vi "Barcode Detector.vi"() -> ()   [LabVIEW 2017]
uses:
  IMAQCV/PIIO.lvlib
  IMAQCV/GPIO/GPIO Pins.ctl
  IMAQCV/IMAQCV.lvlib
  IMAQCV/LVOpenCV.lvlib
  <vilib>/Platform/TimedLoop/XDataNode/wakeup.ctl
  <vilib>/Platform/TimedLoop/XDataNode/XDNodeRunTimeDep.lvlib
  <vilib>/Platform/TimedLoop/XDataNode/nitl_modes.ctl
  <vilib>/Platform/TimedLoop/XDataNode/timing_clust.ctl
  <vilib>/platform/TimedLoop/XDataNode/XDataNode.xnode
  IMAQCV/Support/Camera.ctl
panel:
  out "Barcode":string[](array[string])
  out "output per minute":u32
  in  "FPS":i32=30
  in  "RGB LED 8x8":u32[][](array[colorbox])=[[0, 0, 16777215, 16777215, 16777215, 16777215, 16777215, 16777215], [0, 16777215, 16777215, 16777215, 16777215, 16777215, 16777215, 16777215], [16777215, 16777215, 16777215, 16777215, 16777215, 16777215, 16777215, 16777215], [16777215, 16777215, 0, 0, 0, 0, 0, 0], [16777215, 16777215, 0, 0, 0, 0, 0, 0], [16777215, 16777215, 0, 0, 0, 0, 0, 0], [16777215, 16777215, 0, 0, 0, 0, 0, 0], [0, 16777215, 16777215, 16777215, 16777215, 0, 0, 0]]
  in  "PIN":u8(ring)=23 items=["DIO9"=19, "DIO10"=18, "DIO11"=17, "DIO12"=16, "DIO13"=15, "DIO14"=14, "DIO15"=21, "DIO16"=20, "DIO17"=0, "DIO18"=1, "DIO19"=2, "DIO20"=3, "DIO21"=5, "DIO22"=6, "DIO23"=9, "SDA"=22, "SCL"=23]
  in  "camera input":T1=enum."USB1"
  in  "Image Size":T2(ring)=enum."640 (H)   x  480 (V) "
  out "picture":picture
  out "image processing time (ms)":u32
  out "IO8":bool
  out "IO7":bool
  out "IO6":bool
  out "IO5":bool
  out "IO4":bool
  out "IO3":bool
  out "IO2":bool
  in  "delay (ms)":u32=150
  out "moving time (ms)":u32
  in  "LED Flash":bool
  in  "LED":bool
  in  "Gain (0=auto)":i32(slide) scale=0.0..100.0
  in  "Brightness":i32(slide)=50 scale=0.0..100.0
  in  "Contrast":i32(slide)=50 scale=0.0..100.0
  in  "Saturation":i32(slide)=50 scale=0.0..100.0
  in  "Sharpness":i32(slide)=50 scale=0.0..100.0
  in  "Rotation":i32(ring) items=["0", "90", "180", "270"]
  in  "Flip Horizontal":bool
  in  "Flip Vertical":bool
  in  "AWB":T3(ring)
  in  "Meter":enum16{"AVERAGE", "SPOT", "BACKLIT", "MATRIX"}(ring)
  in  "Effect":T4(ring)
  in  "Shutter (us, 0=auto)":i32
  out "IO1":bool
  in  "stop":bool
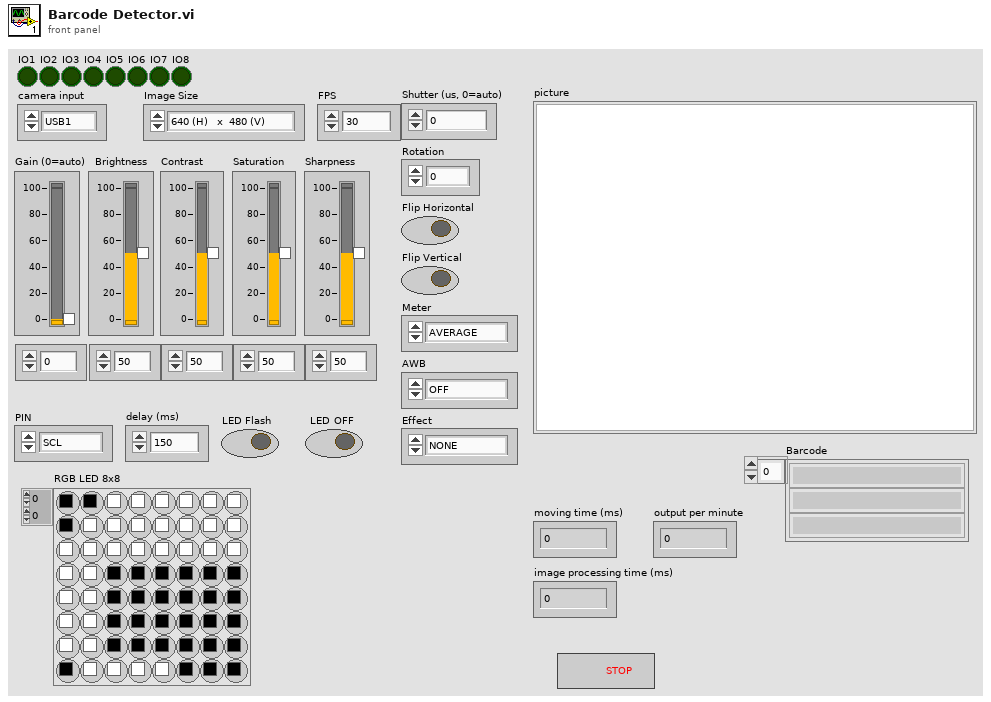
[diagram p1: front panel]
types:
  T1 = typedef "IMAQCV.lvlib/Camera.ctl" = enum8{"Picam", "USB1", "USB2", "USB3", "USB4"}
  T2 = enum16{"320 (H)   x  240 (V)", "352(H)    x  288 (V)", "640 (H)   x  480 (V) ", "800 (H)   x  600 (V)", "1024 (H) x  768 (V)", "1280 (H) x  720 (V)", "1280 (H) x  960 (V)", "1280 (H) x 1024 (V)", "1920 (H) x 1080 (V)"}
  T3 = enum16{"OFF", "AUTO", "SUNLIGHT", "CLOUDY", "SHADE", "TUNGSTEN", "FLUORESCENT", "INCANDESCENT", "FLASH"}
  T4 = enum16{"NONE", "NEGATIVE", "SOLARIZE", "SKETCH", "DENOISE", "EMBOSS", "OILPAINT", "HATCH", "GPEN", "PASTEL", "WATERCOLOR", "FILM", "BLUR", "SATURATION", "COLORSWAP", "WASHEDOUT", "POSTERISE", "COLORPOINT", "COLORBALANCE", "CARTOON"}
  T5 = typedef "Image Type" = u32
  T6 = typedef "PIIO.lvlib/GPIO Pins.ctl" = u8
  T7 = cluster{"GPIO":T6[], "MODE":enum8{"INPUT", "OUTPUT", "PWM_OUTPUT", "GPIO_CLOCK", "SOFT_PWM_OUTPUT", "SOFT_TONE_OUTPUT", "PWM_TONE_OUTPUT"}[]}
  T8 = typedef "IMAQCV.lvlib/IMAQCV Image.ctl" = refnum<vi>
  T9 = typedef "XDNodeRunTimeDep.lvlib/timing_clust.ctl" = cluster{"Expected End [f-1]":u64, "Actual End [f-1]":u64, "Finished Late? [f-1]":bool, "Expected End [i-1]":u64, "Actual End [i-1]":u64, "Finished Late? [i-1]":bool, "Expected Start [i]":u64, "Actual Start [i]":u64, "Expected Start [f]":u64, "Actual Start [f]":u64, "Source Name":string, "Structure Name":string, "Period":i64, "Deadline":i64, "Offset":i64, "Start":i64, "Priority":i32, "Timeout":i32, "Mode":T10, "Wakeup Reason":T11, "Error":errorcluster, "Source Type":string, "Secondary Source Type":string, "Global End Time":u64, "Global Start Time":u64, "Frame Duration":u64, "Iteration Duration":u64, "Assigned CPU":i32, "I/O Scan Engine Mode":u32}
  T10 = typedef "XDNodeRunTimeDep.lvlib/nitl_modes.ctl" = enum32{"No Change", "Process missed periods, maintain original phase", "Discard missed periods, maintain original phase", "Process missed periods, ignore original phase", "Discard missed periods, ignore original phase"}
  T11 = typedef "XDNodeRunTimeDep.lvlib/wakeup.ctl" = enum32{"Normal", "Aborted", "Asynchronous wakeup", "Timing source error", "Timed loop error", "Timeout"}
  T12 = typedef "IMAQ Image.ctl" = refnum<image>
  T13 = cluster{"Data":string, "Special Char 1":string, "Special Char 2":string, "Checksum(s)":string, "Barcode Type":u32, "Confidence Level":sgl, "Bounding Box":cluster{"x":sgl, "y":sgl}[]}[]
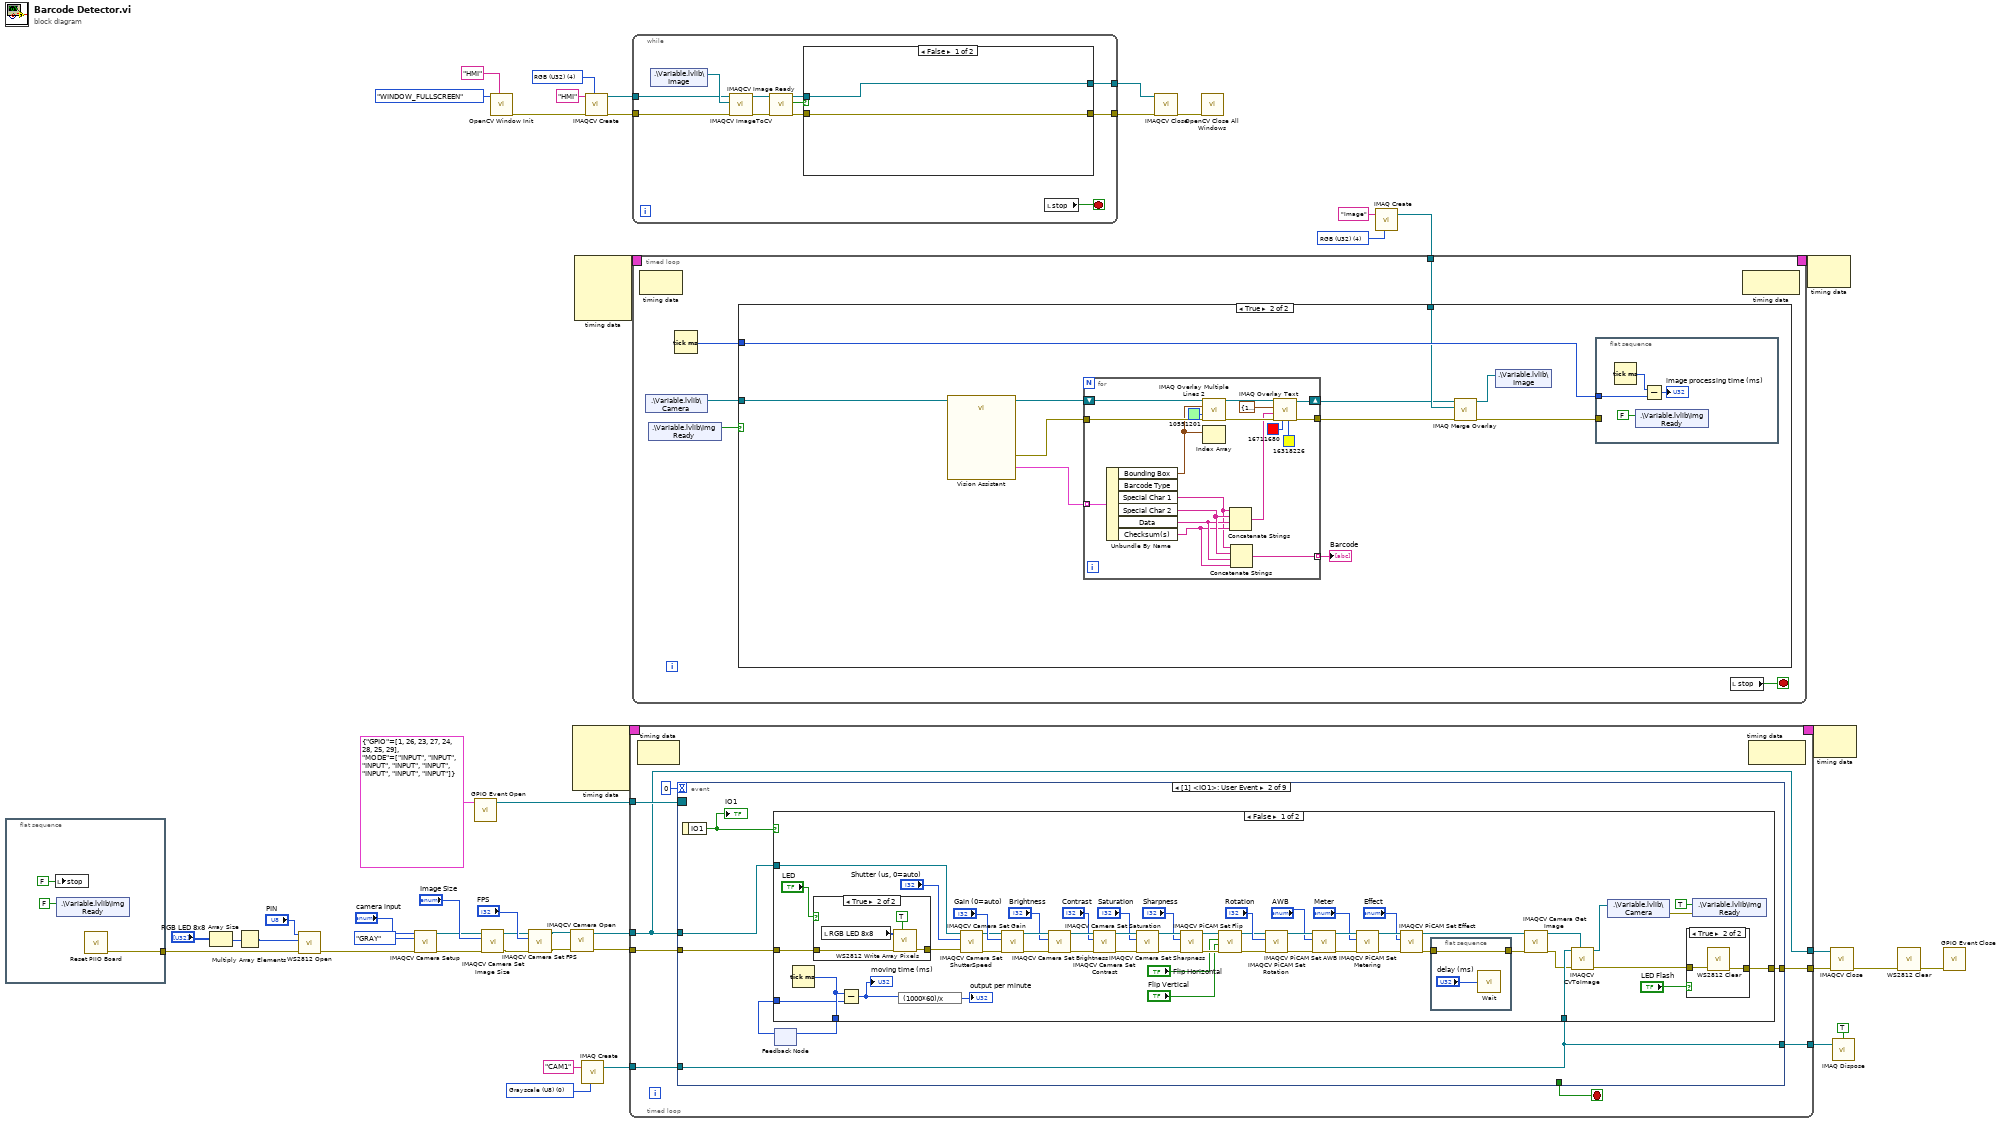
[diagram p0: block diagram]
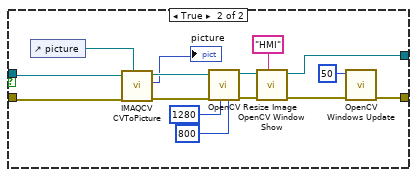
[diagram p2: hidden frame]
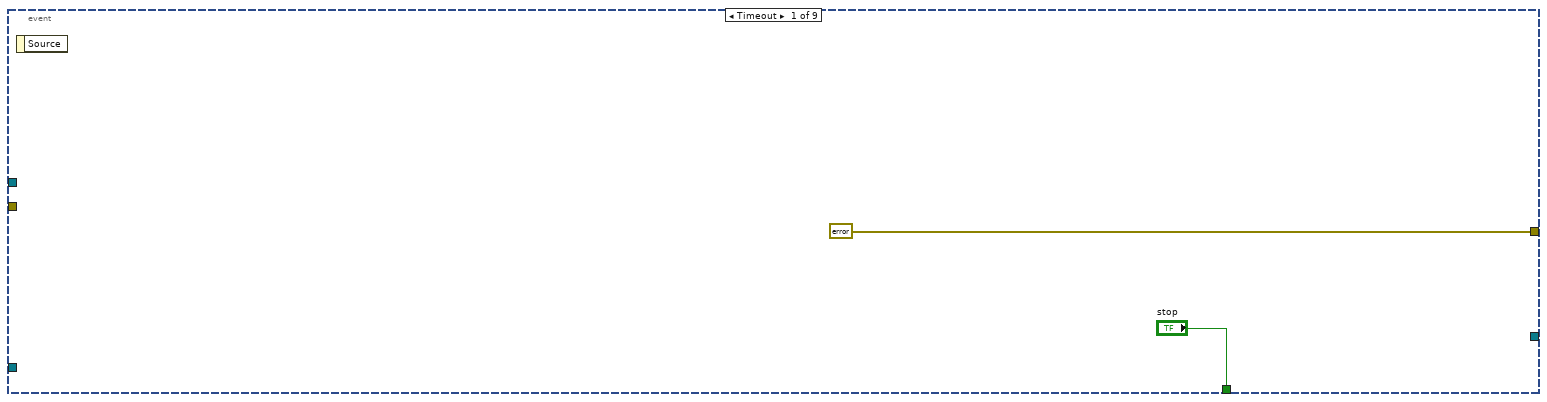
[diagram p4: hidden frame]
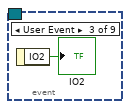
[diagram p8: hidden frame]
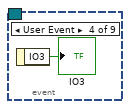
[diagram p9: hidden frame]
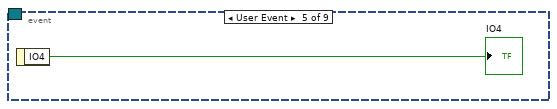
[diagram p10: hidden frame]
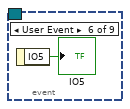
[diagram p11: hidden frame]
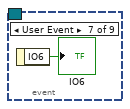
[diagram p12: hidden frame]
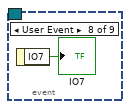
[diagram p13: hidden frame]
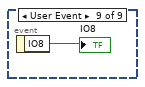
[diagram p14: hidden frame]
diagram:
  w20 = T5 4 items=["Grayscale (U8)", "Grayscale (I16)", "Grayscale (SGL)", "Complex (CSG)", "RGB (U32)", "HSL (U32)", "RGB (U64)", "Grayscale (U16)"] ("Image Type")
  w31 = u32 4 items=["Grayscale (U8)", "Grayscale (I16)", "Grayscale (SGL)", "Complex (CSG)", "RGB (U32)", "HSL (U32)", "RGB (U64)", "Grayscale (U16)"] ("Image Type")
  w36 = T5 0 items=["Grayscale (U8)", "Grayscale (I16)", "Grayscale (SGL)", "Complex (CSG)", "RGB (U32)", "HSL (U32)", "RGB (U64)", "Grayscale (U16)"] ("Image Type")
  n1 = flat-sequence {
    tunnel: [w47] -> w10
    frame #0 {
      n2 = local write "stop"(FALSE ("stop")) -> ()
      n3 = shared-variable ".\\Variable.lvlib\\Img Ready"(FALSE ("outReady")) -> ()  [unwired: 1 in, 1 out]
      n4 = call "Reset PIIO Board.vi"() -> ("error out"=w47:errorcluster)  [unwired: 11 in]
    }
  }
  n5 = Array Size(array="RGB LED 8x8") -> (size(s)=w9:i32[])
  n6 = Multiply Array Elements(1:w9) -> (0:w7:i32)
  n7 = call "WS2812 Open.vi"("Error In"=w10, "Number of LEDs"=w7, "PIN"="PIN") -> ("Error Out"=w25:errorcluster)  [unwired: 8 in]
  n8 = call "IMAQCV Camera Setup.vi"("error in (no error)"=w25, "type"=enum16{"GRAY", "COLOR"}."GRAY", 11:"camera input") -> ("error out"=w26:errorcluster, "image out"=w27:T8)  [unwired: 7 in]
  n9 = call "GPIO Event Open.vi"("GPIO"=T7 {"GPIO"=[1, 26, 23, 27, 24, 28, 25, 29], "MODE"=[enum."INPUT", enum."INPUT", enum."INPUT", enum."INPUT", enum."INPUT", enum."INPUT", enum."INPUT", enum."INPUT"]}) -> ("Event Registration Refnum"=w11:refnum<event-registration>)  [unwired: 9 in, 1 out]
  n10 = call "IMAQCV Camera Set Image Size.vi"("error in (no error)"=w26, "Image Size"="Image Size", "image in"=w27) -> ("error out"=w6:errorcluster, "image out"=w5:T8)  [unwired: 7 in]
  n11 = call "OpenCV Window Init.vi"("window name"="HMI", "mode"=enum8{"WINDOW_AUTOSIZE", "WINDOW_FULLSCREEN"}."WINDOW_FULLSCREEN") -> ("error out"=w16:errorcluster)  [unwired: 9 in]
  n12 = call "IMAQCV Camera Set FPS.vi"("error in (no error)"=w6, "FPS"="FPS", "image in"=w5) -> ("error out"=w4:errorcluster, "image out"=w3:T8)  [unwired: 7 in]
  n13 = call "IMAQCV Camera Open.vi"("error in (no error)"=w4, "image in"=w3) -> ("error out"=w15:errorcluster, "image out"=w14:T8)  [unwired: 8 in]
  n14 = node-c288() -> (w46:T9)  [unwired: 4 in]
  n15 = node-c288() -> (w44:T9)  [unwired: 4 in]
  n16 = call "IMAQ Create"("Image Name"="CAM1", "Image Type"=w36) -> ("New Image"=w35:T12)  [unwired: 3 in, 1 out]
  n17 = call "IMAQCV Create.vi"("Image Type"=w31, "error in (no error)"=w16, "Image Name"="HMI") -> ("error out"=w17:errorcluster, "Image Out"=w19:T8)  [unwired: 7 in]
  n18 = timed-loop {
    tunnel: w11 -> [w55]
    tunnel: [w54] -> w40
    tunnel: w15 -> [w53]
    tunnel: w14 -> [w52]
    tunnel: [w52] -> w38
    tunnel: w35 -> [w51]
    timing: w46 -> [_]
    timing-out: [_] -> w45
    tunnel: [w50] -> w1
    stop <- w57 stop-if-true
    n19 = node-c288() -> ()  [unwired: 1 in, 1 out]
    n20 = event shown="[1] <IO1>: User Event" {
      selector: w55 -> [_ _ _ _ _ _ _ _ _]
      dyn-events: _ -> [_ _ _ _ _ _ _ _ _]
      timeout: 0 -> [_ _ _ _ _ _ _ _ _]
      tunnel: ["stop" _ _ _ _ _ _ _ _] -> w57
      tunnel: [errorcluster {"status"=FALSE, "code"=0, "source"=""} ("error out") w67 _ _ _ _ _ _ _] -> w54
      tunnel: w52 -> [_ w66 _ _ _ _ _ _ _]
      tunnel: w53 -> [_ w68 _ _ _ _ _ _ _]
      tunnel: w51 -> [_ w63 _ _ _ _ _ _ _]
      tunnel: [_ w63 _ _ _ _ _ _ _] -> w50
      event Timeout {
        n21 = event-data() -> ()  [unwired: 1 in, 1 out]
      }
      event User Event {
        n22 = event-data() -> ("IO1"=w62:bool)  [unwired: 1 in]
        "IO1" <- w62
        n23 = feedback #1() -> (w64:u32)  [unwired: 1 in]
        n24 = case shown="False" w62 {
          tunnel: w68 -> [w108 w132]
          tunnel: [w119 w132] -> w67
          tunnel: w66 -> [w72 _]
          tunnel: w63 -> [w111 _]
          tunnel: w64 -> [w114 w131]
          tunnel: [w115 w131] -> w65
          frame False {
            n25 = Tick Count (ms)() -> (millisecond timer value=w115:u32)
            n26 = case shown="True" "LED" {
              tunnel: w108 -> [w121 w125]
              tunnel: [w121 w122] -> w74
              frame False {
              }
              frame True {
                n27 = local read "RGB LED 8x8"() -> (w123:u32[][])
                n28 = call "WS2812 Write Array Pixels.vi"("Refresh? (True)"=TRUE, "Error In"=w125, "pixmap"=w123) -> ("Error Out"=w122:errorcluster)  [unwired: 8 in]
              }
            }
            n29 = Subtract(x=w115, y=w114) -> (x-y=w70:u32)
            "moving time (ms)" <- w70
            n30 = expression code="(1000*60)/x"(w70) -> (→"output per minute":u32)
            n31 = call "IMAQCV Camera Set ShutterSpeed.vi"("error in (no error)"=w74, "shutter speed (us, 0=auto)"="Shutter (us, 0=auto)", "image in"=w72) -> ("error out"=w77:errorcluster, "image out"=w76:T8)  [unwired: 7 in]
            n32 = call "IMAQCV Camera Set Gain.vi"("error in (no error)"=w77, "gain (0=auto)"="Gain (0=auto)", "image in"=w76) -> ("error out"=w105:errorcluster, "image out"=w106:T8)  [unwired: 7 in]
            n33 = call "IMAQCV Camera Set Brightness.vi"("error in (no error)"=w105, "brightness"="Brightness", "image in"=w106) -> ("error out"=w104:errorcluster, "image out"=w101:T8)  [unwired: 7 in]
            n34 = call "IMAQCV Camera Set Contrast.vi"("error in (no error)"=w104, "contrast"="Contrast", "image in"=w101) -> ("error out"=w103:errorcluster, "image out"=w100:T8)  [unwired: 7 in]
            n35 = call "IMAQCV Camera Set Saturation.vi"("error in (no error)"=w103, "saturation"="Saturation", "image in"=w100) -> ("error out"=w102:errorcluster, "image out"=w99:T8)  [unwired: 7 in]
            n36 = call "IMAQCV Camera Set Sharpness.vi"("error in (no error)"=w102, "sharpness"="Sharpness", "image in"=w99) -> ("error out"=w92:errorcluster, "image out"=w91:T8)  [unwired: 7 in]
            n37 = call "IMAQCV PiCAM Set Flip.vi"("error in (no error)"=w92, "vertical"="Flip Vertical", "horizontal"="Flip Horizontal", "image in"=w91) -> ("error out"=w90:errorcluster, "image out"=w89:T8)  [unwired: 6 in]
            n38 = call "IMAQCV PiCAM Set Rotation.vi"("error in (no error)"=w90, "Rotation"="Rotation", "image in"=w89) -> ("error out"=w86:errorcluster, "image out"=w85:T8)  [unwired: 7 in]
            n39 = call "IMAQCV PiCAM Set AWB.vi"("error in (no error)"=w86, "AWB"="AWB", "image in"=w85) -> ("error out"=w83:errorcluster, "image out"=w81:T8)  [unwired: 7 in]
            n40 = call "IMAQCV PiCAM Set Metering.vi"("error in (no error)"=w83, "mode"="Meter", "image in"=w81) -> ("error out"=w82:errorcluster, "image out"=w80:T8)  [unwired: 7 in]
            n41 = call "IMAQCV PiCAM Set Effect.vi"("error in (no error)"=w82, "effect"="Effect", "image in"=w80) -> ("error out"=w73:errorcluster, "image out"=w71:T8)  [unwired: 7 in]
            n42 = flat-sequence {
              tunnel: [w129] -> w120
              tunnel: w73 -> [w129]
              frame #0 {
                n43 = call "Wait"("Count(mSec)"="delay (ms)") -> ()  [unwired: 1 out]
              }
            }
            n44 = call "IMAQCV Camera Get Image.vi"("error in (no error)"=w120, "image in"=w71) -> ("error out"=w110:errorcluster, "image out"=w109:T8)  [unwired: 8 in]
            n45 = call "IMAQCV CVToImage.vi"("cvimage in"=w109, "error in (no error)"=w110, "Variant In"=w111) -> ("error out"=w116:errorcluster, "Variant Out"=w112:refnum<image>)  [unwired: 7 in]
            n46 = shared-variable ".\\Variable.lvlib\\Camera"(w112) -> (error out=w117:errorcluster)  [unwired: 1 in]
            n47 = case shown="True" "LED Flash" {
              tunnel: [w126 w128] -> w119
              tunnel: w116 -> [w126 w127]
              frame False {
              }
              frame True {
                n48 = call "WS2812 Clear.vi"("Error In"=w127) -> ("Error Out"=w128:errorcluster)  [unwired: 10 in]
              }
            }
            n49 = shared-variable ".\\Variable.lvlib\\Img Ready"(TRUE ("ready"), error in=w117) -> ()  [unwired: 1 out]
          }
          frame True {
          }
        }
        n50 = feedback-in #1(w65) -> ()
      }
      event User Event {
        n51 = event-data() -> ("IO2"=→"IO2":bool)  [unwired: 1 in]
      }
      event User Event {
        n52 = event-data() -> ("IO3"=→"IO3":bool)  [unwired: 1 in]
      }
      event User Event {
        n53 = event-data() -> ("IO4"=→"IO4":bool)  [unwired: 1 in]
      }
      event User Event {
        n54 = event-data() -> ("IO5"=→"IO5":bool)  [unwired: 1 in]
      }
      event User Event {
        n55 = event-data() -> ("IO6"=→"IO6":bool)  [unwired: 1 in]
      }
      event User Event {
        n56 = event-data() -> ("IO7"=→"IO7":bool)  [unwired: 1 in]
      }
      event User Event {
        n57 = event-data() -> ("IO8"=→"IO8":bool)  [unwired: 1 in]
      }
    }
    n58 = node-c288() -> ()  [unwired: 1 in, 1 out]
  }
  n59 = while {
    tunnel: [w149] -> w24
    tunnel: [w148] -> w23
    tunnel: w19 -> [w143]
    tunnel: w17 -> [w140]
    stop <- w150 stop-if-true
    n60 = shared-variable ".\\Variable.lvlib\\Image"() -> (w144:refnum<image>)  [unwired: 1 in, 1 out]
    n61 = call "IMAQCV ImageToCV.vi"("error in (no error)"=w140, "Variant In"=w144, "CV in"=w143) -> ("error out"=w141:errorcluster, "CV out"=w142:T8)  [unwired: 7 in]
    n62 = call "IMAQCV Image Ready.vi"("error in (no error)"=w141, "image in"=w142) -> ("error out"=w146:errorcluster, "ready?"=w145:bool, "image out"=w147:T8)  [unwired: 7 in]
    n63 = case shown="False" w145 {
      tunnel: [w151 w164] -> w149
      tunnel: [w152 w163] -> w148
      tunnel: w147 -> [w151 w155]
      tunnel: w146 -> [w152 w156]
      frame False {
      }
      frame True {
        n64 = control-ref of="picture"() -> (w154:refnum<vi>)
        n65 = call "IMAQCV CVToPicture.vi"("picture ref"=w154, "error in (no error)"=w156, "image"=w155) -> ("error out"=w157:errorcluster, "picture"=→"picture":picture, "image out"=w158:T8)  [unwired: 6 in]
        n66 = call "OpenCV Resize Image.vi"("height"=u32 800, "width"=u32 1280, "error in (no error)"=w157, "image in"=w158) -> ("error out"=w159:errorcluster, "image out"=w160:T8)  [unwired: 6 in]
        n67 = call "OpenCV Window Show.vi"("window name"="HMI", "error in (no error)"=w159, "image in"=w160) -> ("error out"=w165:errorcluster, "image out"=w164:T8)  [unwired: 7 in]
        n68 = call "OpenCV Windows Update.vi"("error in (no error)"=w165, "wait ms"=50) -> ("error out"=w163:errorcluster)  [unwired: 8 in, 1 out]
      }
    }
    n69 = local read "stop"() -> (w150:bool)
  }
  n70 = call "IMAQCV Close.vi"("error in (no error)"=w23, "Image"=w24) -> ("error out"=w33:errorcluster)  [unwired: 9 in]
  n71 = call "OpenCV Close All Windows.vi"("error in (no error)"=w33) -> ()  [unwired: 10 in, 1 out]
  n72 = call "IMAQ Create"("Image Name"="Image", "Image Type"=w20) -> ("New Image"=w2:T12)  [unwired: 3 in, 1 out]
  n73 = timed-loop {
    timing: w44 -> [_]
    timing-out: [_] -> w43
    tunnel: w2 -> [w168]
    stop <- w172 stop-if-true
    n74 = node-c288() -> ()  [unwired: 1 in, 1 out]
    n75 = shared-variable ".\\Variable.lvlib\\Camera"() -> (w170:refnum<image>)  [unwired: 1 in, 1 out]
    n76 = shared-variable ".\\Variable.lvlib\\Img Ready"() -> (w169:bool)  [unwired: 1 in, 1 out]
    n77 = Tick Count (ms)() -> (millisecond timer value=w171:u32)
    n78 = case shown="True" w169 {
      tunnel: w171 -> [_ w185]
      tunnel: w170 -> [_ w177]
      tunnel: w168 -> [_ w184]
      frame False {
      }
      frame True {
        n79 = call "Vision Assistant"("Image In"=w177) -> ("Image Out"=w178:T12, "Barcodes (Barcode Reader 1)"=w175:T13, "error out"=w176:errorcluster)  [unwired: 24 in]
        n80 = for {
          tunnel: w175 -> [w203] mode=indexing
          tunnel: w176 -> [w199]
          tunnel: [w197] -> w181
          tunnel: [w187] -> w179 mode=indexing
          shift-right: [w200] -> w180
          shift-left: w178 -> [w186]
          n81 = Unbundle By Name(w203) -> ("Bounding Box"=w196:cluster{"x":sgl, "y":sgl}[], "Special Char 1"=w191:string, "Special Char 2"=w194:string, "Data"=w193:string, "Checksum(s)"=w192:string)  [unwired: 1 out]
          n82 = call "IMAQ Overlay Multiple Lines 2"("Image"=w186, "Line End Points"=w196, "Color"=u32 10551201, "error in (no error)"=w199) -> ("Image Out"=w202:T12, "error out"=w198:errorcluster)  [unwired: 10 in]
          n83 = Index Array(array=w196) -> ()  [unwired: 1 in, 1 out]
          n84 = Concatenate Strings(w191, w194, w193, w192) -> (w195:string)
          n85 = Concatenate Strings(w191, w194, w193, w192) -> (w187:string)
          n86 = call "IMAQ Overlay Text"("BG Color (Transparent)"=u32 16318226, "Text Color (black)"=u32 16711680, "error in (no error)"=w198, "String"=w195, "Origin"=cluster{"X":i32, "Y":i32} {"X"=10, "Y"=20}, "Image"=w202) -> ("error out"=w197:errorcluster, "Image Out"=w200:T12)  [unwired: 4 in]
        }
        "Barcode" <- w179
        n87 = call "IMAQ Merge Overlay"("error in (no error)"=w181, "Image Dst"=w184, "Image Src"=w180) -> ("error out"=w182:errorcluster, "Image Dst Out"=w183:T12)  [unwired: 7 in]
        n88 = shared-variable ".\\Variable.lvlib\\Image"(w183) -> ()  [unwired: 1 in, 1 out]
        n89 = flat-sequence {
          tunnel: w185 -> [w206]
          tunnel: w182 -> [_]
          frame #0 {
            n90 = Tick Count (ms)() -> (millisecond timer value=w207:u32)
            n91 = shared-variable ".\\Variable.lvlib\\Img Ready"(FALSE ("outReady")) -> ()  [unwired: 1 in, 1 out]
            n92 = Subtract(x=w207, y=w206) -> (x-y=→"image processing time (ms)":u32)
          }
        }
      }
    }
    n93 = local read "stop"() -> (w172:bool)
    n94 = node-c288() -> ()  [unwired: 1 in, 1 out]
  }
  n95 = node-c288(w43) -> ()  [unwired: 1 out]
  n96 = node-c288(w45) -> ()  [unwired: 1 out]
  n97 = call "IMAQCV Close.vi"("error in (no error)"=w40, "Image"=w38) -> ("error out"=w41:errorcluster)  [unwired: 9 in]
  n98 = call "IMAQ Dispose"("All Images? (No)"=TRUE, "Image"=w1) -> ()  [unwired: 4 in, 1 out]
  n99 = call "WS2812 Clear.vi"("Error In"=w41) -> ("Error Out"=w39:errorcluster)  [unwired: 10 in]
  n100 = call "GPIO Event Close.vi"("error in (no error)"=w39) -> ()  [unwired: 10 in, 1 out]
